vi "Alert.vi"(5 "error in (no error)":errorcluster) -> (19 "error out":errorcluster)   [LabVIEW 2020]
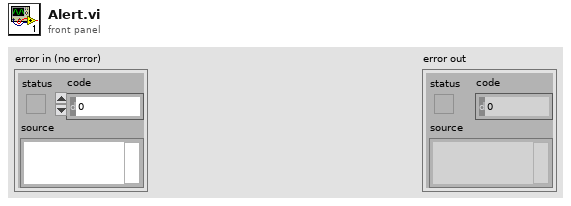
[diagram p1: front panel]
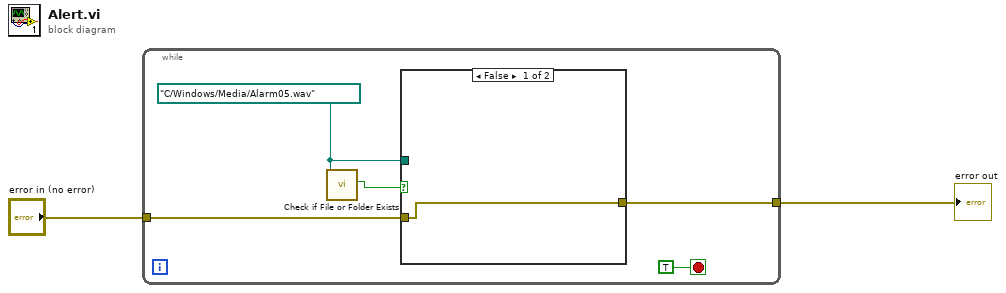
[diagram p0: block diagram]
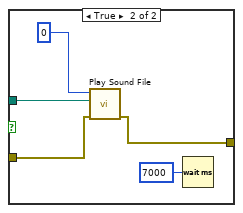
[diagram p2: hidden frame]
diagram:
  n1 = while {
    tunnel: "error in (no error)" -> [w5]
    tunnel: [w4] -> w1
    stop <- TRUE stop-if-true
    w6 = path "C:/Windows/Media/Alarm05.wav"
    n2 = call <vilib>:"Check if File or Folder Exists.vi"("path"=w6) -> ("file or folder exists?"=w3:bool)  [unwired: 8 in, 2 out]
    n3 = case shown="False" w3 {
      tunnel: w6 -> [_ w11]
      tunnel: w5 -> [w8 w10]
      tunnel: [w8 w9] -> w4
      frame False {
      }
      frame True {
        n4 = call <vilib>:"Play Sound File.vi"("error in (no error)"=w10, "path"=w11, "device ID"=u32 0) -> ("error out"=w9:errorcluster)  [unwired: 7 in, 1 out]
        n5 = Wait (ms)(milliseconds to wait=u32 7000) -> ()  [unwired: 1 out]
      }
    }
  }
  "error out" <- w1
